vi "solar_cfg Read (Str).vi"(0 "Config Refnum":refnum<data-value>, 1 "Section":string, 2 "Comment":string, 5 "Key":string, 7 "Value in":string, 9 "Add Quotes? (T)":bool=TRUE, 11 "error in (no error)":errorcluster, 13 "Write If Not Found? (T)":bool=TRUE) -> (4 "dup Config Refnum":refnum<data-value>, 6 "Value out (quotes removed)":string, 10 "Found?":bool, 15 "error out":errorcluster)   [LabVIEW 2018]
doc: "Reads a value associated with a key in a specified section from the configuration file. If the key does not exist and Write If Not Found is True, the VI creates the key in the file. Set a Comment (#...) to add a description after the key's value.\n\n[Section]\nKey = \"Value\" #Comment"
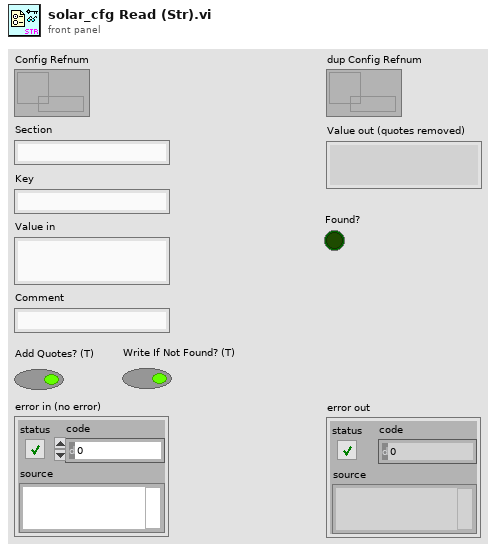
[diagram p1: front panel]
types:
  T1 = cluster{"Dirty":bool, "Semaphore":refnum<queue>, "Sections":cluster{"Section":string, "kvc":string[][]}[], "Path":path}
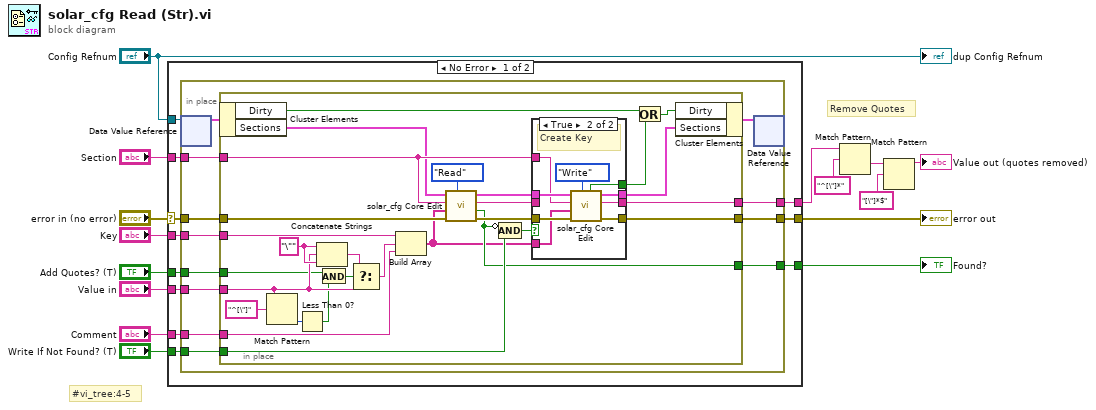
[diagram p0: block diagram]
diagram:
  # "#vi_tree:4-5"
  # "Remove Quotes"
  n1 = case shown="No Error" "error in (no error)" {
    selector: "error in (no error)" -> [w24 w80]
    tunnel: "Config Refnum" -> [w16 _]
    tunnel: "Key" -> [w22 _]
    tunnel: [w25 w80] -> w13
    tunnel: "Section" -> [w23 _]
    tunnel: [w19 _] -> w11
    tunnel: "Value in" -> [w21 w79]
    tunnel: [w18 w79] -> w3
    tunnel: "Comment" -> [w20 _]
    tunnel: "Write If Not Found? (T)" -> [w26 _]
    tunnel: "Add Quotes? (T)" -> [w17 _]
    frame No Error {
      n2 = in-place {
        in-place-border: w26 -> [w38]
        in-place-border: [w37] -> w25
        in-place-border: w24 -> [w36]
        in-place-border: w23 -> [w35]
        in-place-border: w22 -> [w34]
        in-place-border: w21 -> [w33]
        in-place-border: w20 -> [w32]
        in-place-border: [w31] -> w19
        in-place-border: [w30] -> w18
        in-place-border: w17 -> [w27]
        n3 = in-place-dvr #1(w16) -> (w29:T1)  [unwired: 1 out]
        n4 = in-place {
          in-place-border: w38 -> [w65]
          in-place-border: [w63] -> w37
          in-place-border: w36 -> [w62]
          in-place-border: w35 -> [w60]
          in-place-border: w34 -> [w59]
          in-place-border: w33 -> [w44]
          in-place-border: w32 -> [w58]
          in-place-border: [w56] -> w31
          in-place-border: [w53] -> w30
          in-place-border: w27 -> [w40]
          w47 = "\"" ("string")
          n5 = in-place-cluster #2(w29) -> ("Dirty"=w52:bool, "Sections"=w51:cluster{"Section":string, "kvc":string[][]}[])
          n6 = Match Pattern(string=w44, regular expression="^[\"]") -> (offset past match=w42:i32)  [unwired: 1 in, 3 out]
          n7 = Less Than 0?(x=w42) -> (x < 0?=w41:bool)
          n8 = Concatenate Strings(w47, w44, w47) -> (w46:string)
          n9 = And(x=w40, y=w41) -> (x .and. y?=w39:bool)
          n10 = Select(t=w46, s=w39, f=w44) -> (s? t:f=w45:string)
          n11 = Build Array(w59, w45, w58) -> (w55:string[])
          n12 = call "solar_cfg Core Edit.vi"("Action (Read)"=enum8{"Read", "Write", "Parse", "Build"}."Read", "error in (no error)"=w62, "kvc in"=w55, "Section/String in"=w60, "Sections in"=w51) -> ("error out"=w57:errorcluster, "Found?"=w56:bool, "Value/String out"=w54:string, "Sections out"=w66:cluster{"Section":string, "kvc":string[][]}[])  [unwired: 2 in, 1 out]
          n13 = Compound Arithmetic op=AND(invert w56, w65) -> (w64:bool)
          n14 = case "Not Found & Create?" shown="True" w64 {
            tunnel: w66 -> [w67 w78]
            tunnel: w57 -> [w69 w75]
            tunnel: [w69 w74] -> w63
            tunnel: w60 -> [_ w77]
            tunnel: w55 -> [_ w73]
            tunnel: w54 -> [w68 _]
            tunnel: [w68 w72] -> w53
            tunnel: [w67 w71] -> w49
            tunnel: [_ w70] -> w48
            frame False {
            }
            frame True {
              # "Create Key"
              n15 = call "solar_cfg Core Edit.vi"("Action (Read)"=enum8{"Read", "Write", "Parse", "Build"}."Write", "error in (no error)"=w75, "kvc in"=w73, "Section/String in"=w77, "Sections in"=w78) -> ("error out"=w74:errorcluster, "Value/String out"=w72:string, "Sections out"=w71:cluster{"Section":string, "kvc":string[][]}[], "Dirty?"=w70:bool)  [unwired: 2 in, 1 out]
            }
          }
          n16 = Or(x=w52, y=w48) -> (x .or. y?=w50:bool)
          n17 = in-place-cluster #2("Dirty"=w50, "Sections"=w49) -> (w28:T1)
        }
        n18 = in-place-dvr #1(w28) -> ()  [unwired: 2 out]
      }
    }
    frame Error {
    }
  }
  "error out" <- w13
  "Found?" <- w11
  n19 = Match Pattern(string=w3, regular expression="^[\"]*") -> (after substring=w4:string)  [unwired: 1 in, 3 out]
  n20 = Match Pattern(string=w4, regular expression="[\"]*$") -> (before substring=→"Value out (quotes removed)":string)  [unwired: 1 in, 3 out]
  "dup Config Refnum" <- "Config Refnum"
